vi "Day 7 Puzzle 1.vi"(11 "Path":path) -> (3 "Array":cluster{string, i32}[](array[cluster]))   [LabVIEW 2021]
uses:
  <vilib>/Utility/file.llb/Read Delimited Spreadsheet (string).vi
panel:
  out "sum":i32
  out "Second or\n third word":string[](array[string])
  out "First word":string[](array[string])
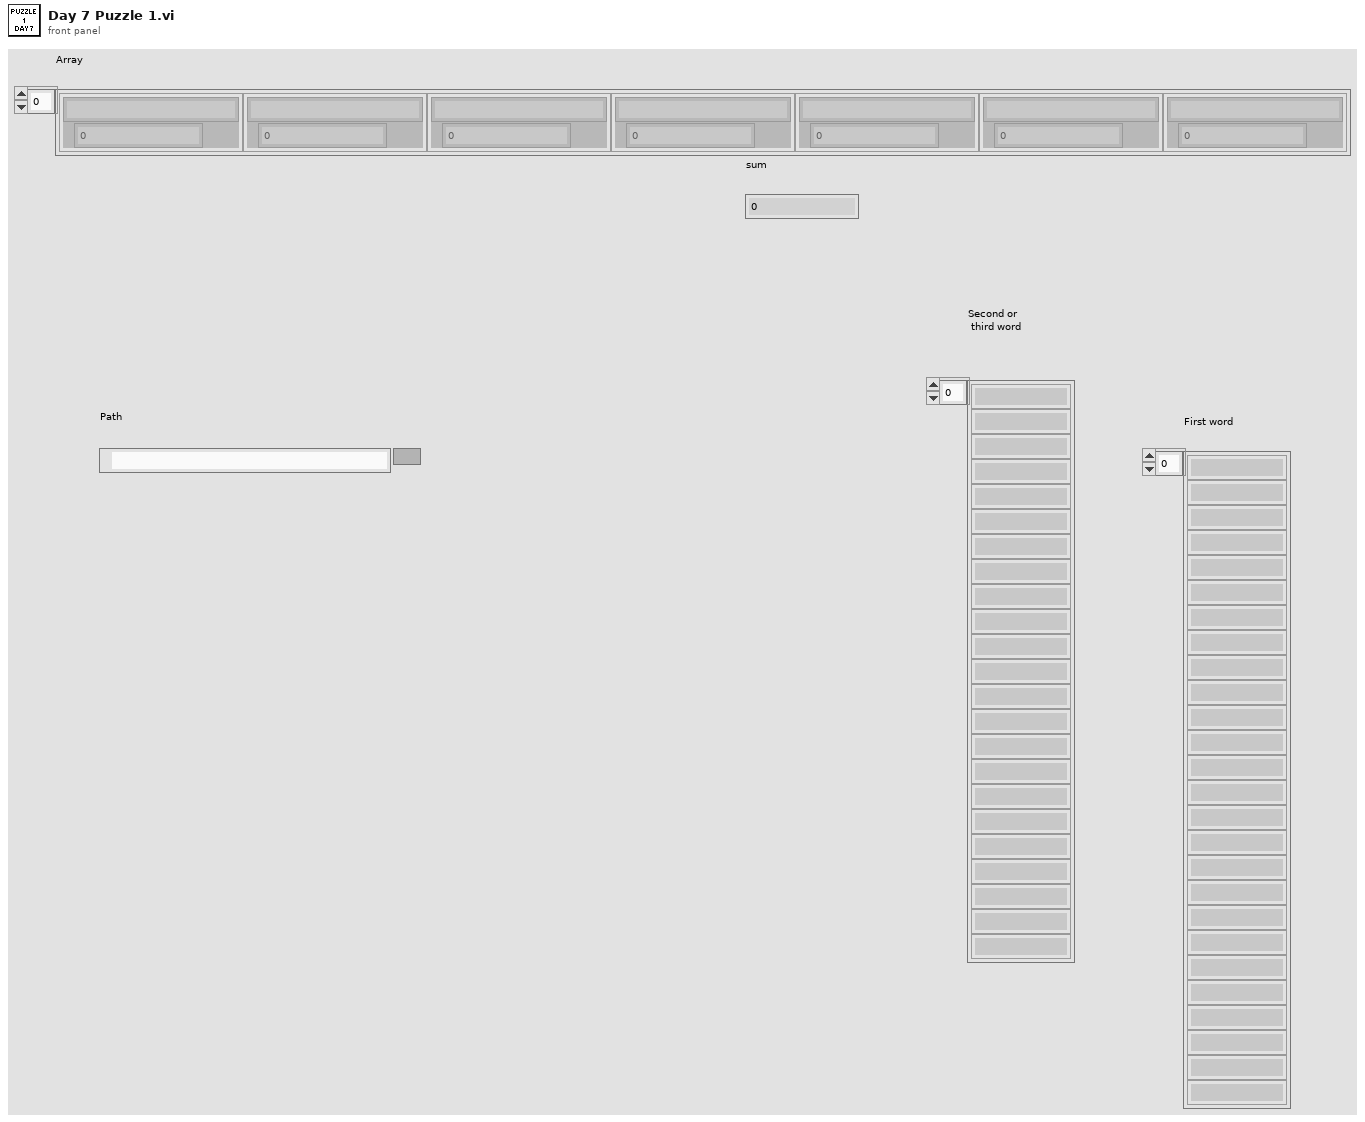
[diagram p1: front panel]
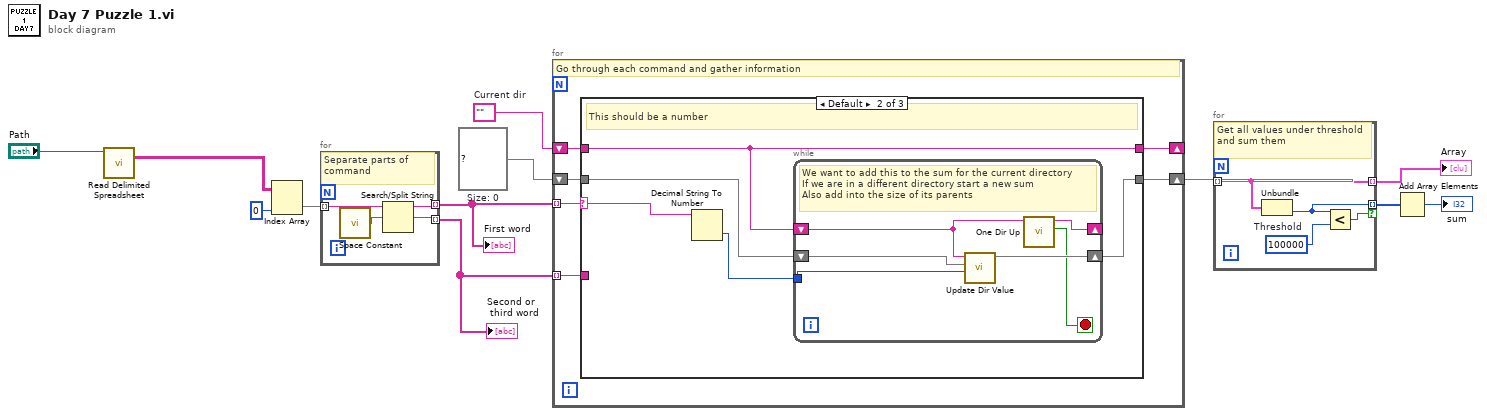
[diagram p0: block diagram]
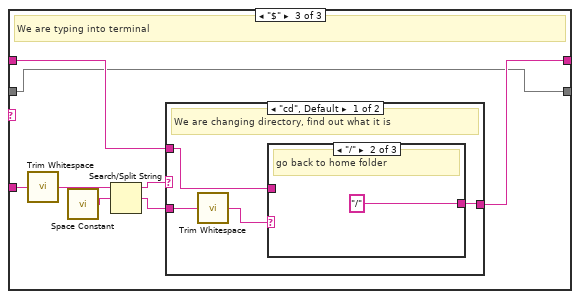
[diagram p3: hidden frame]
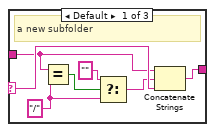
[diagram p4: hidden frame]
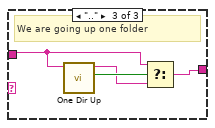
[diagram p5: hidden frame]
diagram:
  w5 = map{string, i32} {}  # Size: 0
  w6 = ""  # Current dir
  n1 = call-poly <vilib>:"Read Delimited Spreadsheet.vi"("file path (dialog if empty)"="Path") -> ("all rows"=w11:string[][])  [unwired: 9 in, 5 out]
  n2 = Index Array(array=w11, index (col)=0 ("disabled index (col)")) -> (element=w9:string[])  [unwired: 1 in]
  n3 = for {
    tunnel: w9 -> [w16] mode=indexing
    tunnel: [w14] -> w8 mode=indexing
    tunnel: [w13] -> w7 mode=indexing
    # "Separate parts of command"
    n4 = call <vilib>:"Space Constant.vi"() -> ("String"=w15:string)
    n5 = Search/Split String(string=w16, search string/char (-)=w15) -> (substring before match=w14:string, match + rest of string=w13:string)  [unwired: 1 in, 1 out]
  }
  "First word" <- w8
  "Second or\n third word" <- w7
  n6 = for {
    tunnel: w8 -> [w22] mode=indexing
    tunnel: w7 -> [w21] mode=indexing
    shift-right: [w19] -> _
    shift-left: w6 -> [w20]
    shift-right: [w17] -> w4
    shift-left: w5 -> [w18]
    # "Go through each command and gather information"
    n7 = case shown="Default" w22 {
      selector: w22 -> [_ w29 _]
      tunnel: w21 -> [_ _ w42]
      tunnel: w20 -> [w24 w27 w38]
      tunnel: [w24 w27 w37] -> w19
      tunnel: w18 -> [w23 w28 w36]
      tunnel: [w23 w26 w36] -> w17
      frame "dir" {
        # "It tells us which directories are contained in current one but because we yet don't know their contents we need to go into those first"
        # "This is a directory, for now this doesn't do anything unless we go in it"
      }
      frame Default {
        # "This should be a number"
        n8 = Decimal String To Number(string=w29) -> (number=w25:i32)  [unwired: 2 in, 1 out]
        n9 = while {
          shift-right: [w32] -> w26
          shift-left: w28 -> [w35]
          shift-right: [w34] -> _
          shift-left: w27 -> [w33]
          tunnel: w25 -> [w31]
          stop <- w30 stop-if-true
          # "We want to add this to the sum for the current directory\nIf we are in a different directory start a new sum\nAlso add into the size of its parents"
          n10 = call "Update Dir Value.vi"("Value"=w31, "Map in"=w35, "Current dir"=w33) -> ("Map out"=w32:map{string, i32})  [unwired: 8 in]
          n11 = call "One Dir Up.vi"("Current dir"=w33) -> ("Top Directory?"=w30:bool, "One up dir"=w34:string)  [unwired: 9 in]
        }
      }
      frame "$" {
        # "We are typing into terminal"
        n12 = call <vilib>:"Trim Whitespace.vi"("string"=w42) -> ("trimmed string"=w41:string)  [unwired: 1 in]
        n13 = call <vilib>:"Space Constant.vi"() -> ("String"=w43:string)
        n14 = Search/Split String(string=w41, search string/char (-)=w43) -> (substring before match=w39:string, match + rest of string=w40:string)  [unwired: 1 in, 1 out]
        n15 = case shown="\"cd\", Default" w39 {
          tunnel: w40 -> [w47 _]
          tunnel: w38 -> [w44 w60]
          tunnel: [w45 w60] -> w37
          frame "cd", Default {
            # "We are changing directory, find out what it is"
            n16 = call <vilib>:"Trim Whitespace.vi"("string"=w47) -> ("trimmed string"=w46:string)  [unwired: 1 in]
            n17 = case shown="\"/\"" w46 {
              selector: w46 -> [w54 _ _]
              tunnel: [w53 "/" w56] -> w45
              tunnel: w44 -> [w52 _ w58]
              frame Default {
                w48 = "/"
                # "a new subfolder"
                n18 = Equal?(x=w52, y=w48) -> (x = y?=w51:bool)
                n19 = Select(t="", s=w51, f=w48) -> (s? t:f=w50:string)
                n20 = Concatenate Strings(w52, w50, w54) -> (w53:string)
              }
              frame "/" {
                # "go back to home folder"
              }
              frame ".." {
                # "We are going up one folder"
                n21 = call "One Dir Up.vi"("Current dir"=w58) -> ("Top Directory?"=w59:bool, "One up dir"=w57:string)  [unwired: 9 in]
                n22 = Select(t=w58, s=w59, f=w57) -> (s? t:f=w56:string)
              }
            }
          }
          frame "ls" {
            # "We are just listing contents"
          }
        }
      }
    }
  }
  n23 = for {
    tunnel: [w64] -> w3 mode=indexing
    tunnel: w4 -> [w64] mode=indexing
    tunnel: [w62] -> w2 mode=indexing if=w61
    w63 = 100000  # Threshold
    # "Get all values under threshold and sum them"
    n24 = Unbundle(w64) -> (w62:i32)  [unwired: 1 out]
    n25 = Less?(x=w62, y=w63) -> (x < y?=w61:bool)
  }
  "Array" <- w3
  n26 = Add Array Elements(numeric array=w2) -> (sum=→"sum":i32)
